vi "Decay data normalizer.vi"(0 "Number of samples":i32=1, 7 "Raw summed data Array":dbl[][](array[numeric]) format="%.2f") -> (8 "Normalized Decay":dbl[](array[numeric]) format="%.2f")   [LabVIEW 2016]
doc: "This subvi normalizes an exponential decay curve\n\nPaul K Dixon\nPhysics 350\nCSUSB Physics"
uses:
  <vilib>/Analysis/baseanly.llb/Mean (DBL).vi
  <vilib>/Analysis/NI_AALBase.lvlib
panel:
  # "Decay Normalizer"
  # "Raw baseline"
  # "Raw decay"
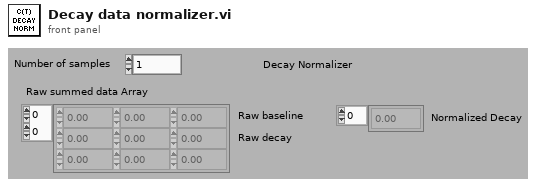
[diagram p1: front panel]
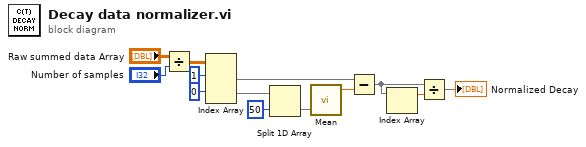
[diagram p0: block diagram]
diagram:
  n1 = Divide(x="Raw summed data Array", y="Number of samples") -> (x/y=w7:dbl[][])
  n2 = Index Array(array=w7, index (row) #1=1 ("Index (row)"), index (row) #2=0 ("Index (row)")) -> (element #1=w12:dbl[], element #2=w2:dbl[])  [unwired: 2 in]
  n3 = Split 1D Array(array=w2, index=50 ("Array Length")) -> (second subarray=w3:dbl[])  [unwired: 1 out]
  n4 = call-poly <vilib>:"Mean.vi"("X"=w3) -> ("mean"=w1:dbl)  [unwired: 1 out]
  n5 = Subtract(x=w12, y=w1) -> (x-y=w10:dbl[])
  n6 = Index Array(array=w10) -> (element=w11:dbl)  [unwired: 1 in]
  n7 = Divide(x=w10, y=w11) -> (x/y=→"Normalized Decay":dbl[])
